vi "Simulation Configuration from Command-Line.vi"(8 "error in":errorcluster, 11 "simulation configuration in":T1={"maxTime"=5.0, "enableVisualization"=TRUE, "Environment Definition"=path "iRobot Navigation State Machine.vi", "Record Location"=path "Simulation Record.xml", "autograde?"=TRUE, "interactive?"=FALSE, "Feedback Mode"=enum."debug navigation", "Robot State Charts"=[path "C:/Users/blueuser/Desktop/Robo Sim Berkley/cpsgrader-release-0.4/Simulators/EECS149lab/src/LabVIEW/statechart/Simulation Statechart.vi"], "statechart"=path "C:/Users/blueuser/Desktop/Robo Sim Berkley/cpsgrader-release-0.4/Simulators/EECS149lab/src/LabVIEW/statechart/Simulation Statechart.vi"}) -> (0 "error out":errorcluster, 3 "simulation configuration out":T1={"maxTime"=5.0, "enableVisualization"=TRUE, "Environment Definition"=path "iRobot Navigation State Machine.vi", "Record Location"=path "Simulation Record.xml", "autograde?"=TRUE, "interactive?"=FALSE, "Feedback Mode"=enum."debug navigation", "Robot State Charts"=[path "C:/Users/blueuser/Desktop/Robo Sim Berkley/cpsgrader-release-0.4/Simulators/EECS149lab/src/LabVIEW/statechart/Simulation Statechart.vi"], "statechart"=path "C:/Users/blueuser/Desktop/Robo Sim Berkley/cpsgrader-release-0.4/Simulators/EECS149lab/src/LabVIEW/statechart/Simulation Statechart.vi"})   [LabVIEW 2015]
uses:
  CyberSim interface/Simulation Configuration.ctl
  autograder/feedbackMode.ctl
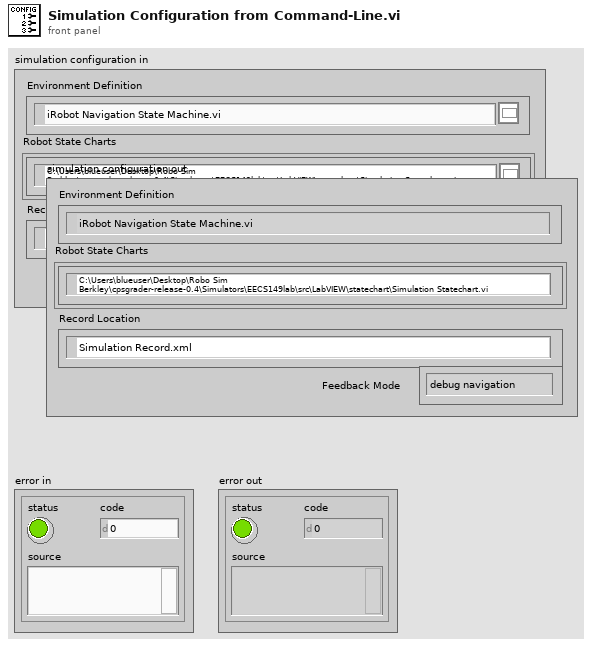
[diagram p1: front panel]
types:
  T1 = typedef "Simulation Configuration.ctl" = cluster{"maxTime":sgl, "enableVisualization":bool, "Environment Definition":path, "Record Location":path, "autograde?":bool, "interactive?":bool, "Feedback Mode":T2, "Robot State Charts":path[], "statechart":path}
  T2 = typedef "feedbackMode.ctl" = enum32{"debug navigation", "debug hill climb", "autograde navigation", "autograde hill climb"}
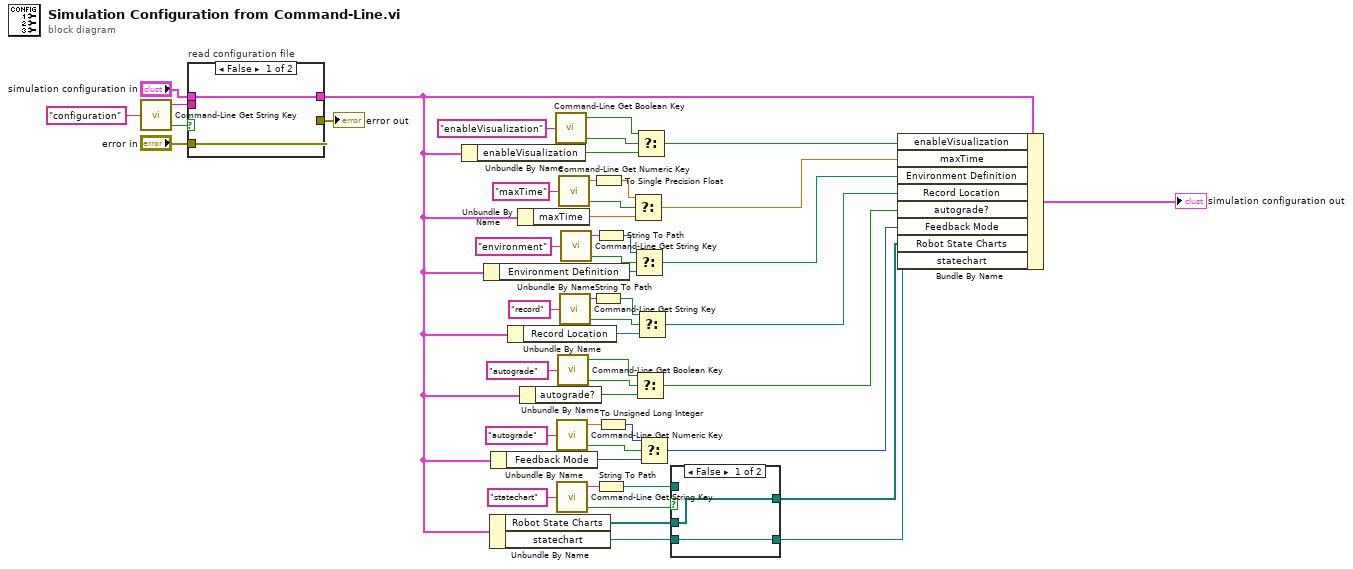
[diagram p0: block diagram]
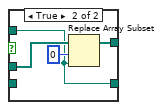
[diagram p2: hidden frame]
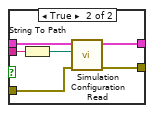
[diagram p3: hidden frame]
diagram:
  n1 = call "Command-Line Get String Key.vi"("string key"="configuration") -> ("key found?"=w45:bool, "string value"=w44:string)  [unwired: 3 in]
  n2 = case "read configuration file" shown="False" w45 {
    tunnel: w44 -> [_ w58]
    tunnel: "simulation configuration in" -> [w52 w55]
    tunnel: [w52 w57] -> w12
    tunnel: "error in" -> [w51 w54]
    tunnel: [w51 w56] -> w21
    frame False {
    }
    frame True {
      n3 = String To Path(string=w58) -> (path=w53:path)
      n4 = call "Simulation Configuration Read.vi"("error in (no error)"=w54, "configuration"=w53, "simulation configuration"=w55) -> ("error out"=w56:errorcluster, "simulation configuration"=w57:T1)  [unwired: 7 in]
    }
  }
  "error out" <- w21
  n5 = Unbundle By Name(w12) -> ("enableVisualization"=w42:bool)
  n6 = Unbundle By Name(w12) -> ("Environment Definition"=w38:path)
  n7 = Unbundle By Name(w12) -> ("Robot State Charts"=w4:path[], "statechart"=w1:path)
  n8 = Unbundle By Name(w12) -> ("Feedback Mode"=w13:T2)
  n9 = Unbundle By Name(w12) -> ("Record Location"=w23:path)
  n10 = Unbundle By Name(w12) -> ("maxTime"=w34:sgl)
  n11 = Unbundle By Name(w12) -> ("autograde?"=w18:bool)
  n12 = call "Command-Line Get Boolean Key.vi"("boolean key"="enableVisualization" ("string key")) -> ("key found?"=w41:bool, "boolean value"=w40:bool)  [unwired: 3 in]
  n13 = call "Command-Line Get Numeric Key.vi"("numeric key"="autograde") -> ("key found?"=w14:bool, "numeric value"=w11:dbl)  [unwired: 3 in]
  n14 = call "Command-Line Get String Key.vi"("string key"="statechart") -> ("key found?"=w6:bool, "string value"=w7:string)  [unwired: 3 in]
  n15 = call "Command-Line Get Boolean Key.vi"("boolean key"="autograde" ("numeric key")) -> ("key found?"=w19:bool, "boolean value"=w17:bool)  [unwired: 3 in]
  n16 = call "Command-Line Get Numeric Key.vi"("numeric key"="maxTime") -> ("key found?"=w33:bool, "numeric value"=w32:dbl)  [unwired: 3 in]
  n17 = call "Command-Line Get String Key.vi"("string key"="record" ("numeric key")) -> ("key found?"=w26:bool, "string value"=w39:string)  [unwired: 3 in]
  n18 = call "Command-Line Get String Key.vi"("string key"="environment" ("numeric key")) -> ("key found?"=w35:bool, "string value"=w37:string)  [unwired: 3 in]
  n19 = String To Path(string=w39) -> (path=w27:path)
  n20 = To Single Precision Float(number=w32) -> (single precision float=w31:sgl)
  n21 = String To Path(string=w37) -> (path=w36:path)
  n22 = String To Path(string=w7) -> (path=w5:path)
  n23 = To Unsigned Long Integer(number=w11) -> (unsigned 32bit integer=w10:u32)
  n24 = Select(t=w31, s=w33, f=w34) -> (s? t:f=w28:sgl)
  n25 = Select(t=w36, s=w35, f=w38) -> (s? t:f=w25:path)
  n26 = Select(t=w17, s=w19, f=w18) -> (s? t:f=w16:bool)
  n27 = Select(t=w40, s=w41, f=w42) -> (s? t:f=w30:bool)
  n28 = Select(t=w27, s=w26, f=w23) -> (s? t:f=w22:path)
  n29 = Select(t=w10, s=w14, f=w13) -> (s? t:f=w9:u32)
  n30 = case shown="False" w6 {
    tunnel: w5 -> [_ w61]
    tunnel: w4 -> [w60 w64]
    tunnel: [w60 w62] -> w3
    tunnel: [w59 w61] -> w2
    tunnel: w1 -> [w59 _]
    frame False {
    }
    frame True {
      n31 = Replace Array Subset(array=w64, new element=w61, index=0) -> (w62:path[])
    }
  }
  n32 = Bundle By Name(cluster=w12, "enableVisualization"=w30, "maxTime"=w28, "Environment Definition"=w25, "Record Location"=w22, "autograde?"=w16, "Feedback Mode"=w9, "Robot State Charts"=w3, "statechart"=w2) -> (→"simulation configuration out":T1)
